vi "I-V analisys.vi"() -> ()   [LabVIEW 2016]
uses:
  <vilib>/Waveform/WDTOps.llb/WDT Get Waveform Subset DBL.vi
  <vilib>/Analysis/NI_AALPro.lvlib
panel:
  out "XY Graph 2":cluster{"Y":dbl[], dbl[]}(graph)
  out "Field":waveform(dbl)(graph)
  in  "Field channel":string="Field"
  out "XY Graph":cluster{"Y":dbl[], "Y":dbl[]}[](graph)
  in  "Stop Button":bool
  out "Waveform Graph":waveform(dbl)[](graph)
  in  "Interval duration":dbl=0.0001 format="%#_6ps"
  in  "Interval start":dbl=-0.009 format="%#_6ps"
  in  "I to V delay":dbl(slide) step=1e-08 scale=5e-08..1e-07 scale format="%#_6ps"
  in  "group name":string="p"
  in  "V channel":string="Va"
  in  "I channel":string="I"
  in  "File Path Control":path=path "\\\\eden\\NHMFLDATA/Data/cell2daq/February_2018/022218/p019_022218.tdms"
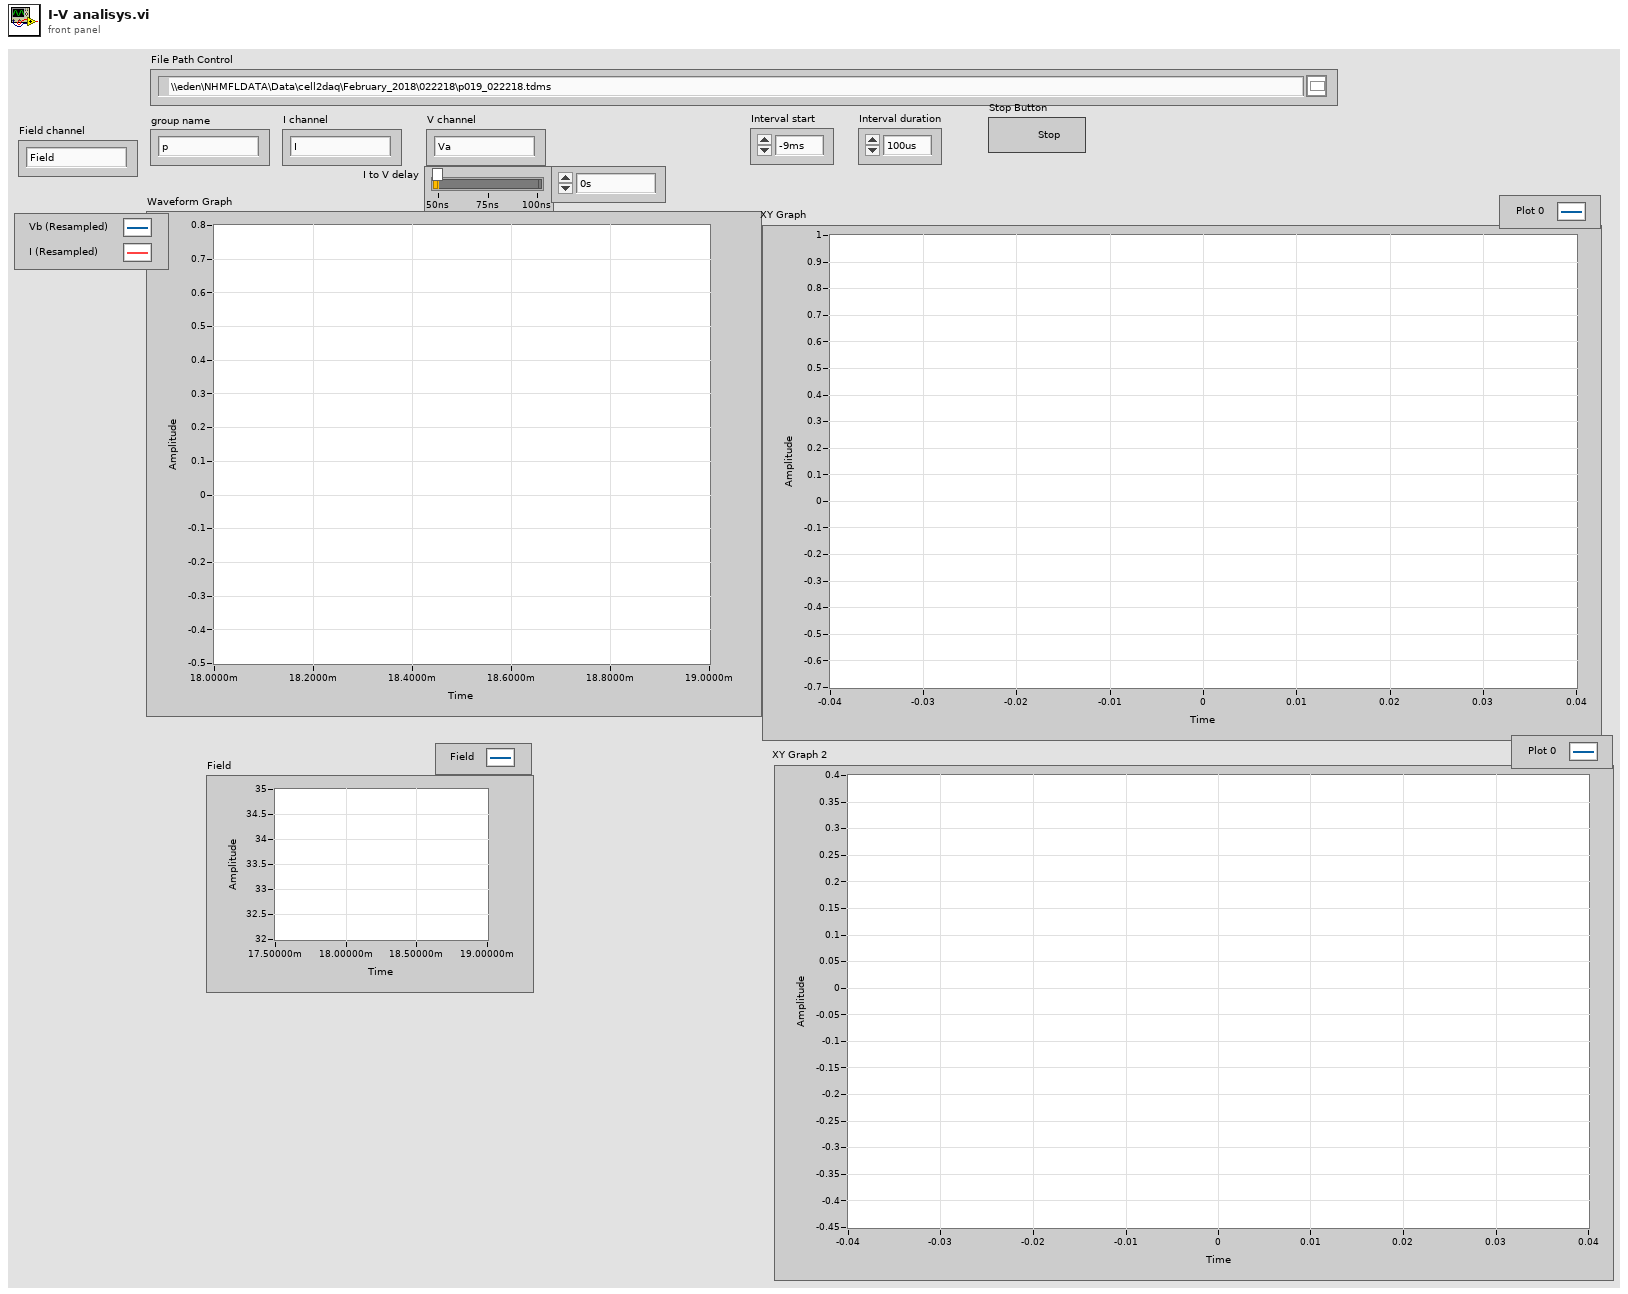
[diagram p1: front panel]
types:
  T1 = enum16{"open", "open or create", "create or replace", "create", "open (read-only)"}
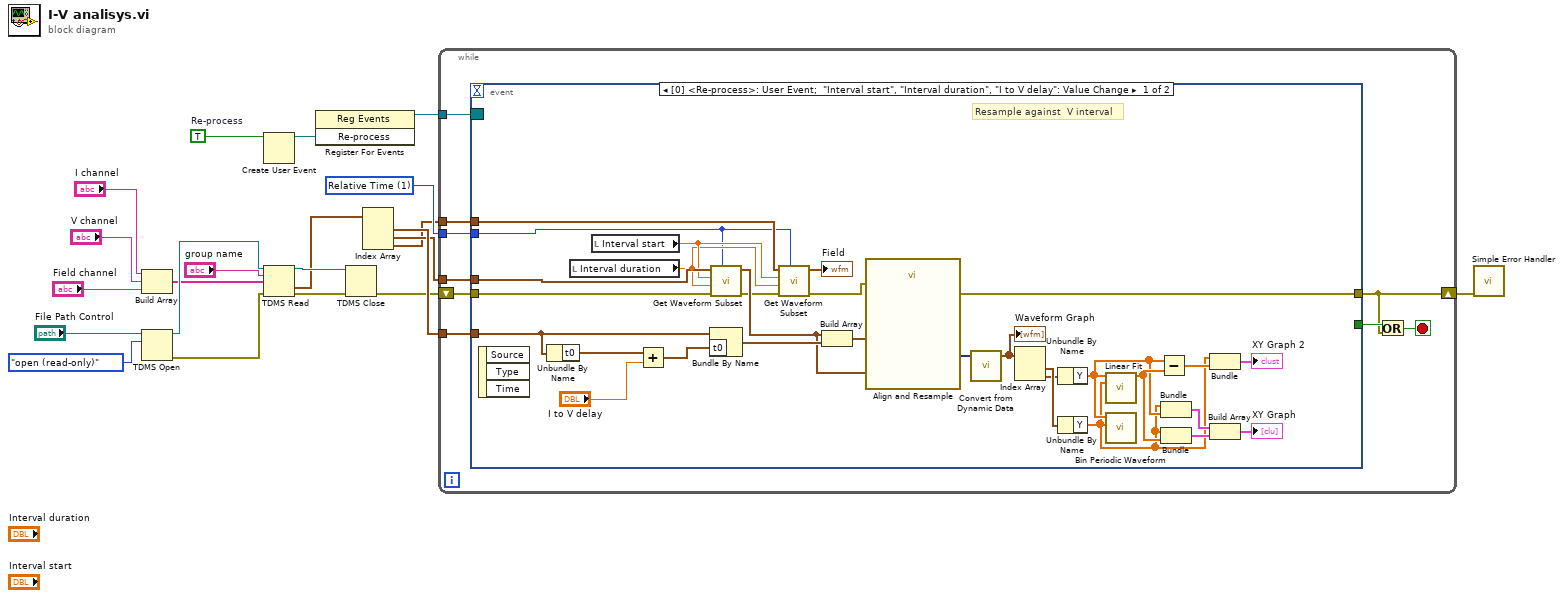
[diagram p0: block diagram]
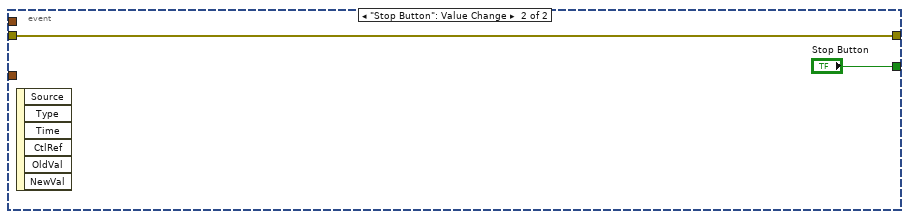
[diagram p2: hidden frame]
diagram:
  w7 = TRUE  # Re-process
  w8 = u16 1 items=["Samples", "Relative Time"] ("start/duration format")
  n1 = Build Array("I channel", "V channel", "Field channel") -> (w14:string[])
  n2 = TDMS Open(10:T1."open (read-only)" ("operation (0:open)"), 11:"File Path Control") -> (0:w17:errorcluster, 3:w19:refnum<k34>)  [unwired: 5 in]
  n3 = Create User Event(user event datatype=w7) -> (user event=w6:refnum<user-event>)  [unwired: 1 in, 1 out]
  n4 = TDMS Read(0:w19, 5:"group name", 7:w14, 11:w17) -> (4:w12:refnum<k34>, 10:w5:waveform(dbl)[], 15:w13:errorcluster)  [unwired: 4 in, 3 out]
  n5 = register-events(w6) -> (reference out=w4:refnum<event-registration>)  [unwired: 2 in, 1 out]
  n6 = TDMS Close(8:w13, 11:w12) -> (0:w9:errorcluster)  [unwired: 1 out]
  n7 = Index Array(array=w5) -> (element #1=w11:waveform(dbl), element #2=w10:waveform(dbl), element #3=w1:waveform(dbl))  [unwired: 3 in]
  n8 = while {
    tunnel: w11 -> [w30]
    tunnel: w10 -> [w29]
    tunnel: w8 -> [w27]
    tunnel: w4 -> [w25]
    shift-right: [w23] -> w3
    shift-left: w9 -> [w28]
    tunnel: w1 -> [w22]
    stop <- w24 stop-if-true
    n9 = event shown="[0] <Re-process>: User Event;  \"Interval start\", \"Interval duration\", \"I to V delay\": Value Change" {
      selector: w25 -> [_ _]
      dyn-events: _ -> [_ _]
      timeout: _ -> [_ _]
      tunnel: w30 -> [w57 _]
      tunnel: w29 -> [w55 _]
      tunnel: w28 -> [w54 w60]
      tunnel: w27 -> [w36 _]
      tunnel: [_ "Stop Button"] -> w26
      tunnel: [w38 w60] -> w23
      tunnel: w22 -> [w43 _]
      event User Event; "Interval start", "Interval duration", "I to V delay": Value Change {
        # "Resample against  V interval"
        n10 = event-data() -> ()  [unwired: 1 in, 3 out]
        n11 = Unbundle By Name(w57) -> ("t0"=w59:timestamp)
        n12 = local read "Interval duration"() -> (w41:dbl)
        n13 = local read "Interval start"() -> (w42:dbl)
        n14 = Add(x=w59, y="I to V delay") -> (x+y=w58:timestamp)
        n15 = Bundle By Name(cluster=w57, "t0"=w58) -> (w53:waveform(dbl))
        n16 = call-poly <vilib>:"Get Waveform Subset.vi"("start/duration format"=w36, "error in (no error)"=w54, "duration"=w41, "start samples/time"=w42, "waveform in"=w55) -> ("error out"=w40:errorcluster, "waveform out"=w51:waveform(dbl))  [unwired: 1 in, 2 out]
        n17 = call-poly <vilib>:"Get Waveform Subset.vi"("start/duration format"=w36, "error in (no error)"=w40, "duration"=w41, "start samples/time"=w42, "waveform in"=w43) -> ("error out"=w39:errorcluster, "waveform out"=→"Field":waveform(dbl))  [unwired: 1 in, 2 out]
        n18 = Build Array(w51, w53) -> (w52:waveform(dbl)[])
        n19 = call "Align and Resample"("Reference Signal"=w51, "error in (no error)"=w39, "Signals"=w52) -> ("error out"=w38:errorcluster, "Resampled Signals"=w56:dynamicdata)  [unwired: 6 in, 1 out]
        n20 = call "Convert from Dynamic Data"("Dynamic Data Type"=w56) -> ("Array of Waveform"=w49:waveform(dbl)[])  [unwired: 3 in]
        "Waveform Graph" <- w49
        n21 = Index Array(array=w49) -> (element #1=w48:waveform(dbl), element #2=w47:waveform(dbl))  [unwired: 2 in]
        n22 = Unbundle By Name(w47) -> ("Y"=w32:dbl[])
        n23 = Unbundle By Name(w48) -> ("Y"=w31:dbl[])
        n24 = call <vilib>:"Linear Fit.vi"("Y"=w32, "X"=w31) -> ("Best Linear Fit"=w35:dbl[])  [unwired: 9 in, 4 out]
        n25 = call "Bin Periodic Waveform.vi"("Y Array"=w31, "X Array"=w32) -> ()  [unwired: 10 in]
        n26 = Subtract(x=w32, y=w35) -> (x-y=w34:dbl[])
        n27 = Bundle("Y"=w31, "Y"=w32) -> (w46:cluster{"Y":dbl[], "Y":dbl[]})  [unwired: 1 in]
        n28 = Bundle("Y"=w31, "Best Linear Fit"=w35) -> (w44:cluster{"Y":dbl[], "Best Linear Fit":dbl[]})  [unwired: 1 in]
        n29 = Bundle("Y"=w31, w34) -> (→"XY Graph 2":cluster{"Y":dbl[], dbl[]})  [unwired: 1 in]
        n30 = Build Array(w46, w44) -> (→"XY Graph":cluster{"Y":dbl[], "Best Linear Fit":dbl[]}[])
      }
      event "Stop Button": Value Change {
        n31 = event-data() -> ()  [unwired: 1 in, 6 out]
      }
    }
    n32 = Or(x=w26, y=w23) -> (x .or. y?=w24:bool)
  }
  n33 = call <vilib>:"Simple Error Handler.vi"("error in (no error)"=w3) -> ()  [unwired: 4 in, 5 out]
